vi "CreateSQLConditionSubVI.vi"(1 "To":timestamp, 2 "From":timestamp, 3 "Conection Type":string) -> (0 "Condition":string)   [LabVIEW 2016]
doc: "Creates an SQL statement to filter the search of the DB"
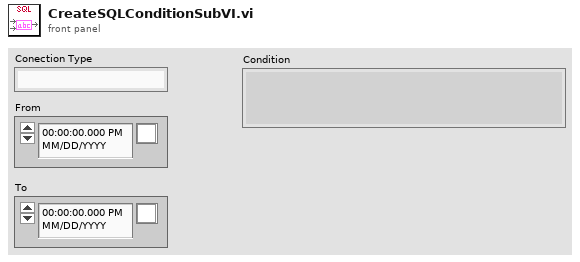
[diagram p1: front panel]
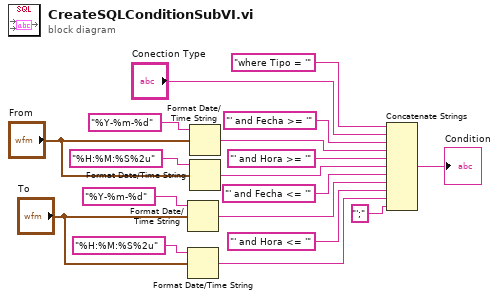
[diagram p0: block diagram]
diagram:
  n1 = Format Date/Time String(time format string (%c)="%Y-%m-%d", seconds (now)="To") -> (date/time string=w3:string)  [unwired: 1 in]
  n2 = Format Date/Time String(time format string (%c)="%H:%M:%S%2u", seconds (now)="To") -> (date/time string=w2:string)  [unwired: 1 in]
  n3 = Format Date/Time String(time format string (%c)="%Y-%m-%d", seconds (now)="From") -> (date/time string=w5:string)  [unwired: 1 in]
  n4 = Format Date/Time String(time format string (%c)="%H:%M:%S%2u", seconds (now)="From") -> (date/time string=w4:string)  [unwired: 1 in]
  n5 = Concatenate Strings("where Tipo = '" ("string"), "Conection Type", "' and Fecha >= '" ("string"), w5, "' and Hora >= '" ("string"), w4, "' and Fecha <= '" ("string"), w3, "' and Hora <= '" ("string"), w2, "';" ("string")) -> (→"Condition":string)
